vi "HDPE Choose Folder.vi"(8 "error in":errorcluster) -> (0 "error Out":errorcluster, 2 "Cancel 2":bool, 3 "Choose the folder path Out":path)   [LabVIEW 2019]
panel:
  in  "Cancel":bool
  in  "Choose the folder path":path
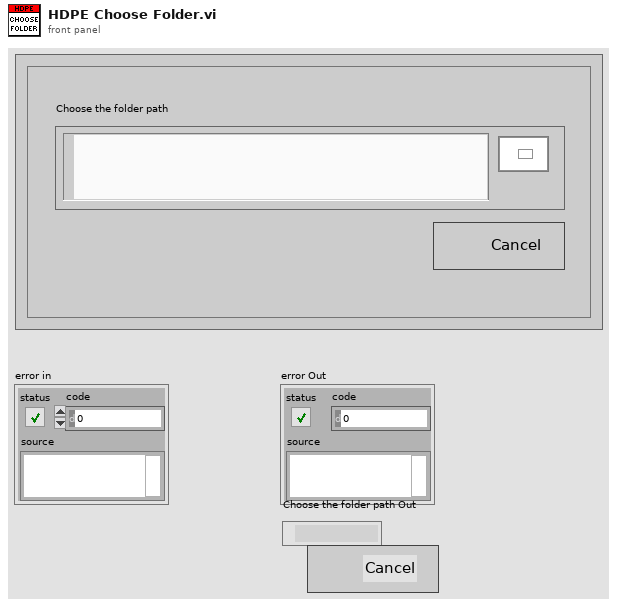
[diagram p1: front panel]
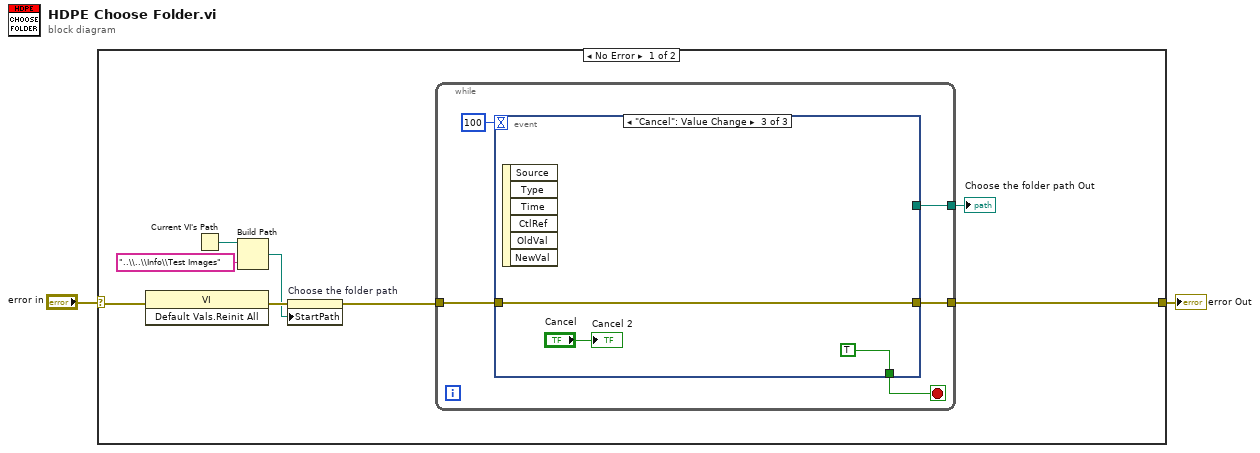
[diagram p0: block diagram]
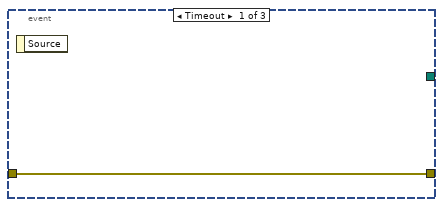
[diagram p2: hidden frame]
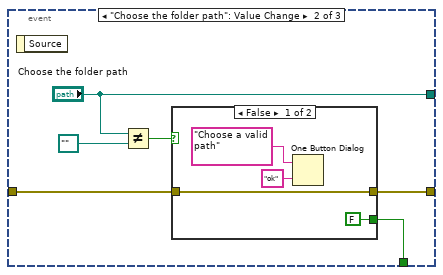
[diagram p3: hidden frame]
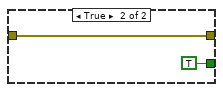
[diagram p4: hidden frame]
diagram:
  n1 = case shown="No Error" "error in" {
    selector: "error in" -> [w9 w32]
    tunnel: [w10 w32] -> w1
    frame No Error {
      n2 = invoke class="VI" method="Default Vals.Reinit All"(error in=w9) -> (error out=w7:errorcluster)  [unwired: 2 in, 2 out]
      n3 = Current VI's Path() -> (path=w5:path)
      n4 = Build Path(base path=w5, name or relative path="..\\..\\Info\\Test Images") -> (appended path=w3:path)
      n5 = property on="Choose the folder path" class="Path"(error in=w7, "StartPath"=w3) -> (error out=w6:errorcluster)  [unwired: 1 in, 1 out]
      n6 = while {
        tunnel: w6 -> [w14]
        tunnel: [w13] -> w10
        tunnel: [w11] -> w8
        stop <- w12 stop-if-true
        n7 = event shown="[2] \"Cancel\": Value Change" {
          selector: _ -> [_ _ _]
          dyn-events: _ -> [_ _ _]
          timeout: 100 -> [_ _ _]
          tunnel: w14 -> [w16 w17 w30]
          tunnel: [w16 w19 w30] -> w13
          tunnel: [_ "Choose the folder path" _] -> w11
          tunnel: [_ w18 TRUE] -> w12
          event Timeout {
            n8 = event-data() -> ()  [unwired: 1 in, 1 out]
          }
          event "Choose the folder path": Value Change {
            n9 = event-data() -> ()  [unwired: 1 in, 1 out]
            n10 = Not Equal?(x="Choose the folder path", y=path "") -> (x != y?=w21:bool)
            n11 = case shown="False" w21 {
              tunnel: w17 -> [w26 w28]
              tunnel: [w26 w28] -> w19
              tunnel: [FALSE TRUE] -> w18
              frame False {
                n12 = One Button Dialog(message="Choose a valid  path", button name ("OK")="ok") -> ()  [unwired: 1 out]
              }
              frame True {
              }
            }
          }
          event "Cancel": Value Change {
            n13 = event-data() -> ()  [unwired: 1 in, 6 out]
            "Cancel 2" <- "Cancel"
          }
        }
      }
      "Choose the folder path Out" <- w8
    }
    frame Error {
    }
  }
  "error Out" <- w1
